vi "On Uninstall of JSONtext.vi"() -> ()   [LabVIEW 2017]
uses:
  <vilib>/Palette API/Palette Menu/Public Type Define/Palette type.ctl
  <vilib>/Palette API/Palette Menu/Public Type Define/Item.ctl
  <vilib>/Palette API/Palette Menu/Palette Menu.lvlib
panel:
  out "error out":errorcluster
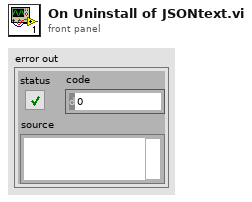
[diagram p1: front panel]
types:
  T1 = typedef "Palette Menu.lvlib/Palette type.ctl" = i32
  T2 = typedef "Palette Menu.lvlib/Palette Data.ctl" = cluster{"display name":string, "view format":T3, "palette width":i16, "items":T4, "256 color icon":picture, "B&W color icon":picture, "help information":T6, "palette description":string, "synchronize information":T7}
  T3 = typedef "Palette Menu.lvlib/View Format.ctl" = u16
  T4 = typedef "Palette Menu.lvlib/Items.ctl" = T5[]
  T5 = typedef "Palette Menu.lvlib/Item.ctl" = cluster{"item path":path, "library path (.lvlib)":path, "use default lvlib palette":bool, "short name":string, "place VI contents":bool, "hide synchronized item":bool, "reserve spot for synch item":bool, "configure when placing VI contents":bool}
  T6 = typedef "Palette Menu.lvlib/Help Info.ctl" = cluster{"help tag":string, "help file path ":path}
  T7 = typedef "Palette Menu.lvlib/Synchronize Info.ctl" = cluster{"synchronize with directory":bool, "synchronize directory path":path}
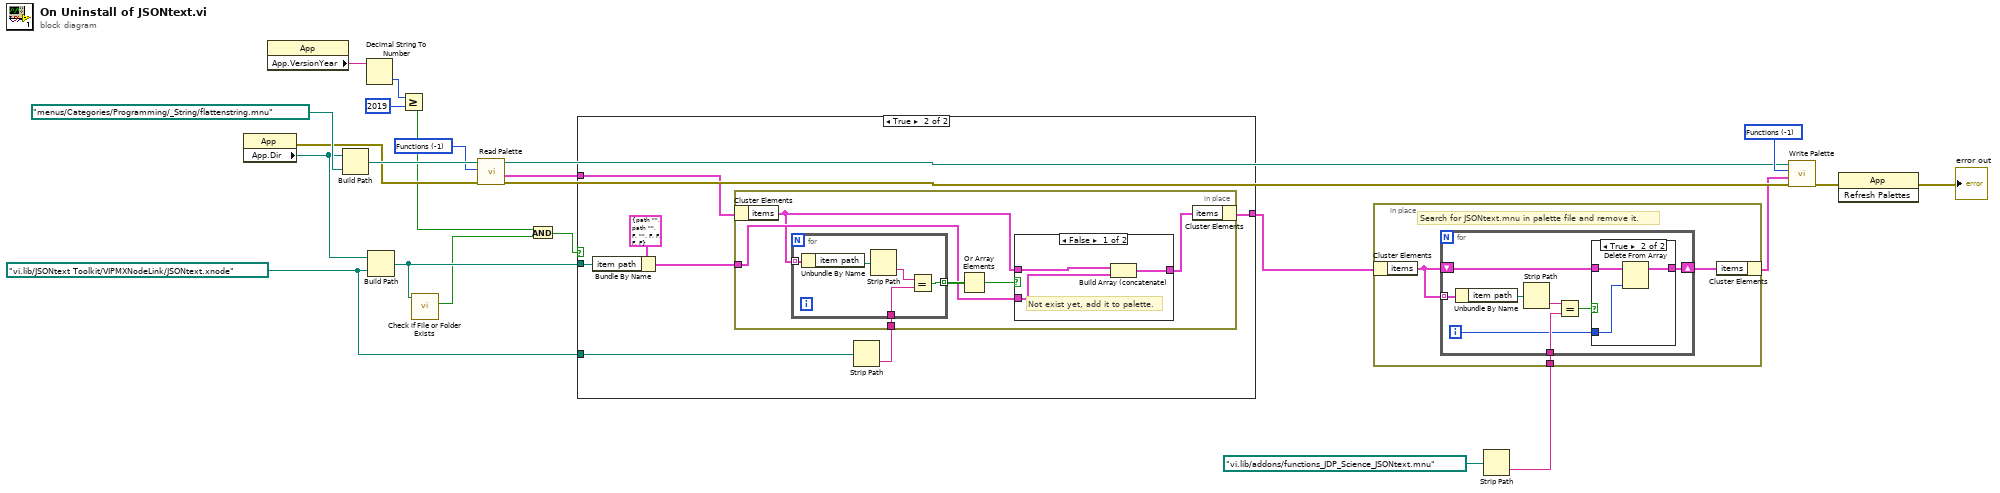
[diagram p0: block diagram]
diagram:
  w8 = T1 -1 items=["Functions"=-1, "Controls"=-2] ("palette type")
  w11 = T1 -1 items=["Functions"=-1, "Controls"=-2] ("palette type")
  w17 = path "vi.lib/JSONtext Toolkit/VIPMXNodeLink/JSONtext.xnode"
  n1 = property class="App"() -> (error out=w18:errorcluster, "App.Dir"=w1:path)  [unwired: 2 in, 1 out]
  n2 = property class="App"() -> ("App.VersionYear"=w21:string)  [unwired: 2 in, 2 out]
  n3 = Build Path(base path=w1, name or relative path=path "menus/Categories/Programming/_String/flattenstring.mnu") -> (appended path=w19:path)
  n4 = Decimal String To Number(string=w21) -> (number=w23:i32)  [unwired: 2 in, 1 out]
  n5 = Build Path(base path=w1, name or relative path=w17) -> (appended path=w16:path)
  n6 = Greater Or Equal?(x=w23, y=2019) -> (x >= y?=w14:bool)
  n7 = call <vilib>:"Check if File or Folder Exists.vi"("path"=w16) -> ("file or folder exists?"=w15:bool)  [unwired: 8 in, 2 out]
  n8 = call <vilib>:"Read Palette.vi"("error in (no error)"=w18, "palette type"=w8, "palette path"=w19) -> ("error out"=w10:errorcluster, "palette data"=w7:T2, "duplicate palette path"=w9:path)  [unwired: 1 in, 5 out]
  n9 = And(x=w14, y=w15) -> (x .and. y?=w6:bool)
  n10 = case shown="True" w6 {
    tunnel: w17 -> [_ w31]
    tunnel: w16 -> [_ w30]
    tunnel: w7 -> [w24 w27]
    tunnel: [w24 w26] -> w5
    frame False {
    }
    frame True {
      n11 = Bundle By Name(cluster=T5 {"item path"=path "", "library path (.lvlib)"=path "", "use default lvlib palette"=FALSE, "short name"="", "place VI contents"=FALSE, "hide synchronized item"=FALSE, "reserve spot for synch item"=FALSE, "configure when placing VI contents"=FALSE} ("Items"), "item path"=w30) -> (w28:T5)
      n12 = Strip Path(path=w31) -> (name=w25:string)  [unwired: 1 out]
      n13 = in-place {
        in-place-border: w28 -> [w34]
        in-place-border: w25 -> [w37]
        n14 = in-place-cluster #1(w27) -> ("items"=w32:T4)
        n15 = for {
          tunnel: w32 -> [w46] mode=indexing
          tunnel: w37 -> [w43]
          tunnel: [w42] -> w36 mode=indexing
          n16 = Unbundle By Name(w46) -> ("item path"=w45:path)
          n17 = Strip Path(path=w45) -> (name=w44:string)  [unwired: 1 out]
          n18 = Equal?(x=w44, y=w43) -> (x = y?=w42:bool)
        }
        n19 = Or Array Elements(Boolean array=w36) -> (logical OR=w35:bool)
        n20 = case shown="False" w35 {
          tunnel: w34 -> [w40 _]
          tunnel: [w39 w41] -> w33
          tunnel: w32 -> [w38 w41]
          frame False {
            # "Not exist yet, add it to palette."
            n21 = Build Array (concatenate)(w38, w40) -> (w39:T4)
          }
          frame True {
            # "Alreay exists on palette,\ndo nothing."
          }
        }
        n22 = in-place-cluster #1("items"=w33) -> (w26:T2)
      }
    }
  }
  n23 = Strip Path(path=path "vi.lib/addons/functions_JDP_Science_JSONtext.mnu" ("name or relative path")) -> (name=w3:string)  [unwired: 1 out]
  n24 = in-place {
    in-place-border: w3 -> [w49]
    # "Search for JSONtext.mnu in palette file and remove it."
    n25 = in-place-cluster #2(w5) -> ("items"=w48:T4)
    n26 = for {
      tunnel: w48 -> [w57] mode=indexing
      tunnel: w49 -> [w54]
      shift-right: [w50] -> w47
      shift-left: w48 -> [w52]
      i -> [w51]
      n27 = Unbundle By Name(w57) -> ("item path"=w56:path)
      n28 = Strip Path(path=w56) -> (name=w55:string)  [unwired: 1 out]
      n29 = Equal?(x=w55, y=w54) -> (x = y?=w53:bool)
      n30 = case shown="True" w53 {
        tunnel: w52 -> [w58 w60]
        tunnel: w51 -> [_ w61]
        tunnel: [w58 w59] -> w50
        frame False {
        }
        frame True {
          n31 = Delete From Array(array=w60, index=w61) -> (array with subset deleted=w59:T4)  [unwired: 1 in, 1 out]
        }
      }
    }
    n32 = in-place-cluster #2("items"=w47) -> (w2:T2)
  }
  n33 = call <vilib>:"Write Palette.vi"("error in (no error)"=w10, "palette data"=w2, "palette type"=w11, "palette path"=w9) -> ("error out"=w13:errorcluster)  [unwired: 1 in, 6 out]
  n34 = invoke class="App" method="Refresh Palettes"(error in=w13) -> (error out=→"error out":errorcluster)  [unwired: 2 in, 2 out]
